vi "problem_2_part2.vi"() -> ()   [LabVIEW 2020]
panel:
  out "Area":dbl
  out "Perimeter":dbl
  in  "Radius of \nthe Circle":dbl format="%#_6f"
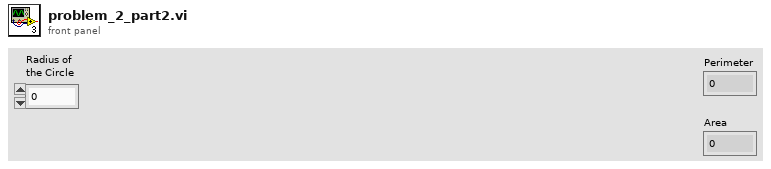
[diagram p1: front panel]
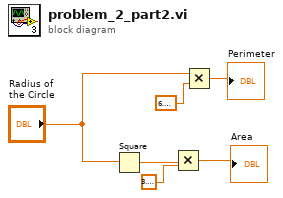
[diagram p0: block diagram]
diagram:
  n1 = Square(x="Radius of \nthe Circle") -> (x^2=w6:dbl)
  n2 = Multiply(x=w6, y=3.141592653589793) -> (x*y=→"Area":dbl)
  n3 = Multiply(x="Radius of \nthe Circle", y=6.283185307179586) -> (x*y=→"Perimeter":dbl)
